vi "Process Data.vi"(7 "AdasLvTemplate in":refnum<class "AdasLvTemplate.lvclass">, 8 "error in":errorcluster, 11 "Node in":refnum<class "AMS Climate Chamber Template.lvclass">) -> (0 "error out":errorcluster, 3 "Node out":refnum<class "AMS Climate Chamber Template.lvclass">, 5 "AdasLvTemplate out":refnum<class "AdasLvTemplate.lvclass">)   [LabVIEW 2023, in "AMS Climate Chamber Template.lvlib" / "AMS Climate Chamber Template.lvclass"]
uses:
  AMS Climate Chamber Template.lvclass
  <vilib>/ADAS Replay HIL/ADAS Plugin Utilities/AdasLvTemplate/AdasLvTemplate.lvclass
  AMS Climate Chamber Template.lvclass/AMS Climate Chamber Template.ctl
  C:/Program Files/National Instruments/AMS plugin/Capabilities/Capabilities/High Level Capabilities/Climate Chamber Cluster/Producer Control.ctl
  C:/Program Files/National Instruments/AMS plugin/Capabilities/Capabilities/High Level Capabilities/Climate Chamber Cluster/Producer Ch.ctl
  C:/Program Files/National Instruments/AMS plugin/Capabilities/Capabilities/High Level Capabilities/Climate Chamber Cluster/Climate Chamber Cluster.lvclass
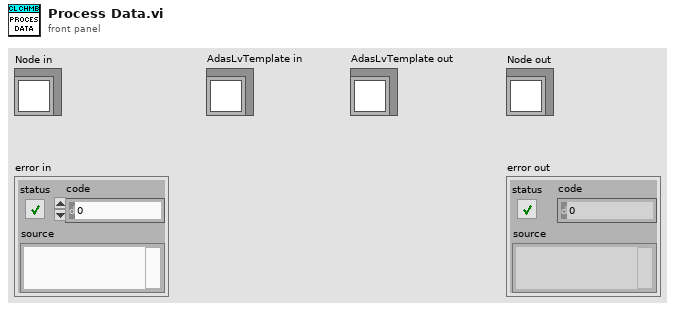
[diagram p1: front panel]
types:
  T1 = typedef "AMS Climate Chamber Template.lvlib/AMS Climate Chamber Template.lvclass/Configuration Params.ctl" = cluster{"Common":T2, "Amount of Channels":u32, "Address":string}
  T2 = typedef "Template Node.lvlib/Template Node.lvclass/Common Configuration Params.ctl" = cluster{"Iteration Interval (s)":dbl, "T0 (ns)":u64, "Priority":i32, "Processor":i32, "Wait in Ready State":bool}
  T3 = typedef "Climate Chamber Cluster.lvclass/Consumer Ch.ctl" = cluster{"Temperature.SP":dbl, "TemperatureMIN.SP":dbl, "TemperatureMAX.SP":dbl, "TemperatureGrad.SP":dbl, "Humidity.SP":dbl, "HumidityMIN.SP":dbl, "HumidityMAX.SP":dbl, "HumidityGrad.SP":dbl}
  T4 = typedef "Climate Chamber Cluster.lvclass/Consumer Control.ctl" = cluster{"OnOff.ACT":bool, "ErrorAcknowledge.ACT":bool}
  T5 = typedef "Climate Chamber Cluster.lvclass/Producer Control.ctl" = cluster{"OnOff.STS":i32, "Error.STS":i32, "Watchdog.STS":i32}
  T6 = typedef "Climate Chamber Cluster.lvclass/Producer Ch.ctl" = cluster{"Temperature.AV":dbl, "Humidity.AV":dbl}
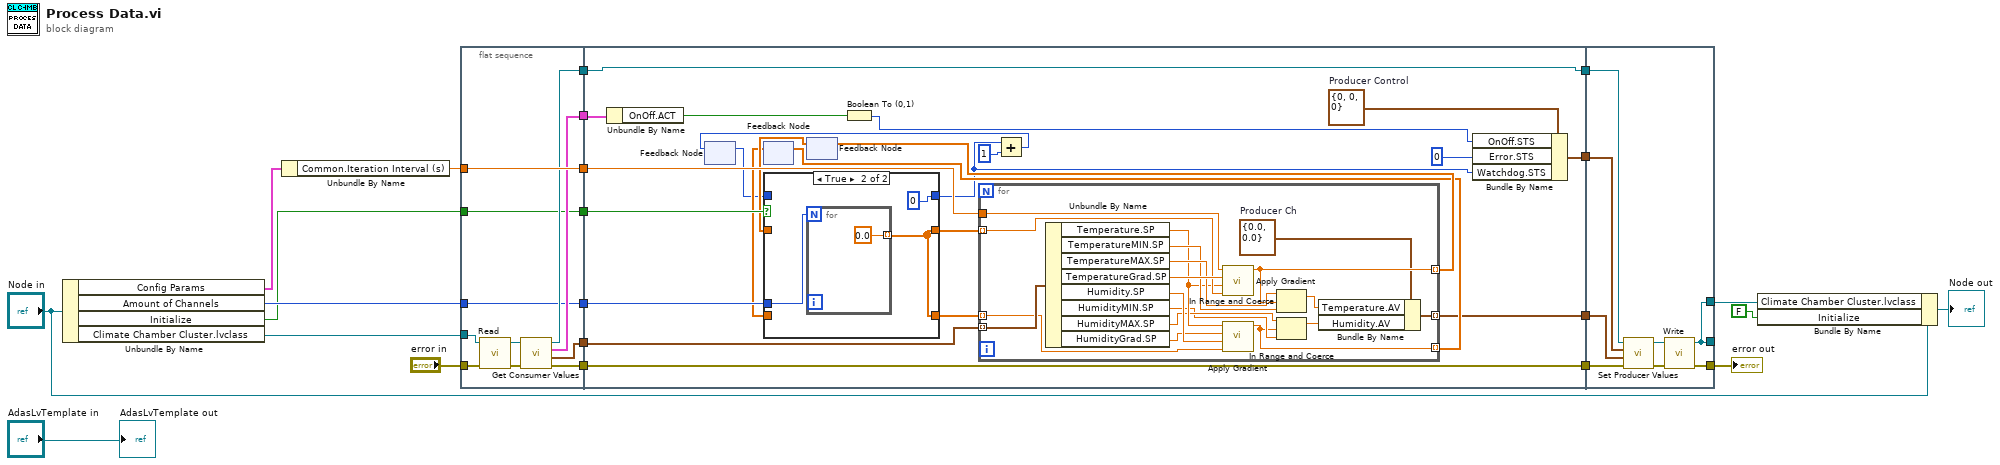
[diagram p0: block diagram]
diagram:
  n1 = Unbundle By Name("Node in") -> ("Config Params"=w22:T1, "Amount of Channels"=w5:u32, "Initialize"=w4:bool, "Climate Chamber Cluster.lvclass"=w1:refnum<class "Climate Chamber Cluster.lvclass">)
  n2 = Unbundle By Name(w22) -> ("Common.Iteration Interval (s)"=w13:dbl)
  n3 = flat-sequence {
    tunnel: w1 -> [w34]
    tunnel: [w28] -> w21
    tunnel: [w31] -> w20
    tunnel: "error in" -> [w33]
    tunnel: [w26] -> w15
    tunnel: [w30] -> w14
    tunnel: w13 -> [w32]
    tunnel: [w32] -> w12
    tunnel: w5 -> [w25]
    tunnel: w4 -> [w24]
    tunnel: [w25] -> w3
    tunnel: [w24] -> w2
    tunnel: w21 -> [w50]
    tunnel: w20 -> [w57]
    tunnel: [w51] -> w19
    tunnel: [w50] -> w18
    tunnel: [w49] -> w16
    tunnel: w15 -> [w49]
    tunnel: w14 -> [w43]
    tunnel: w12 -> [w48]
    tunnel: [w45] -> w11
    tunnel: w3 -> [w42]
    tunnel: w2 -> [w41]
    tunnel: w19 -> [w83]
    tunnel: w18 -> [w85]
    tunnel: w16 -> [w87]
    tunnel: [w90] -> w10
    tunnel: [w89] -> _
    tunnel: w11 -> [w86]
    tunnel: [w89] -> w8
    frame #0 {
      n4 = call-dynamic "Read.vi"("error in"=w33, "Climate Chamber Cluster.lvclass in"=w34) -> ("error out"=w27:errorcluster, "Climate Chamber Cluster.lvclass out"=w29:refnum<class "Climate Chamber Cluster.lvclass">)  [unwired: 8 in]
      n5 = call "Get Consumer Values.vi"("error in"=w27, "Climate Chamber Cluster.lvclass in"=w29) -> ("error out"=w26:errorcluster, "Consumer Ch"=w30:T3[], "Consumer Control"=w31:T4, "Climate Chamber Cluster.lvclass out"=w28:refnum<class "Climate Chamber Cluster.lvclass">)  [unwired: 6 in]
    }
    frame #1 {
      w56 = T5 {"OnOff.STS"=0, "Error.STS"=0, "Watchdog.STS"=0}  # Producer Control
      n6 = Unbundle By Name(w57) -> ("OnOff.ACT"=w55:bool)
      n7 = feedback #1() -> (w35:u16)  [unwired: 1 in]
      n8 = feedback #2() -> (w38:dbl[])  [unwired: 1 in]
      n9 = feedback #3() -> (w40:dbl[])  [unwired: 1 in]
      n10 = case shown="True" w41 {
        tunnel: [w60 w62] -> w39
        tunnel: w42 -> [_ w63]
        tunnel: w40 -> [w60 _]
        tunnel: w38 -> [w59 _]
        tunnel: [w59 w62] -> w37
        tunnel: [w58 u16 0] -> w36
        tunnel: w35 -> [w58 _]
        frame False {
        }
        frame True {
          n11 = for {
            N: w63 -> [_]
            tunnel: [0.0 ("Current Setpoint")] -> w62 mode=indexing
          }
        }
      }
      n12 = Boolean To (0,1)(Boolean=w55) -> (0, 1=w54:i16)
      n13 = for {
        tunnel: w43 -> [w82] mode=indexing
        tunnel: w48 -> [w81]
        tunnel: w39 -> [w77] mode=indexing
        tunnel: [w76] -> w47 mode=indexing
        tunnel: [w70] -> w46 mode=indexing
        tunnel: w37 -> [w69] mode=indexing
        tunnel: [w65] -> w45 mode=indexing
        w68 = T6 {"Temperature.AV"=0.0, "Humidity.AV"=0.0}  # Producer Ch
        n14 = Unbundle By Name(w82) -> ("Temperature.SP"=w73:dbl, "TemperatureMIN.SP"=w78:dbl, "TemperatureMAX.SP"=w79:dbl, "TemperatureGrad.SP"=w80:dbl, "Humidity.SP"=w75:dbl, "HumidityMIN.SP"=w71:dbl, "HumidityMAX.SP"=w72:dbl, "HumidityGrad.SP"=w74:dbl)
        n15 = call "Apply Gradient.vi"("Reminder"=w77, "Setpoint"=w73, "Gradient"=w80, "Iteration Interval"=w81) -> ("Current Setpoint"=w76:dbl)  [unwired: 7 in]
        n16 = call "Apply Gradient.vi"("Reminder"=w69, "Setpoint"=w75, "Gradient"=w74, "Iteration Interval"=w73) -> ("Current Setpoint"=w70:dbl)  [unwired: 7 in]
        n17 = In Range and Coerce(upper limit=w79, x=w76, lower limit=w78) -> (coerced(x)=w67:dbl)  [unwired: 1 out]
        n18 = In Range and Coerce(upper limit=w72, x=w70, lower limit=w71) -> (coerced(x)=w66:dbl)  [unwired: 1 out]
        n19 = Bundle By Name(cluster=w68, "Temperature.AV"=w67, "Humidity.AV"=w66) -> (w65:T6)
      }
      n20 = feedback-in #2(w46) -> ()
      n21 = feedback-in #3(w47) -> ()
      n22 = Add(x=w36, y=u16 1) -> (x+y=w52:u16)
      n23 = feedback-in #1(w52) -> ()
      n24 = Bundle By Name(cluster=w56, "OnOff.STS"=w54, "Error.STS"=0, "Watchdog.STS"=w36) -> (w51:T5)
    }
    frame #2 {
      n25 = call "Set Producer Values.vi"("error in"=w87, "Producer Ch"=w86, "Producer Control"=w83, "Climate Chamber Cluster.lvclass in"=w85) -> ("error out"=w88:errorcluster, "Climate Chamber Cluster.lvclass out"=w84:refnum<class "Climate Chamber Cluster.lvclass">)  [unwired: 6 in]
      n26 = call-dynamic "Write.vi"("error in"=w88, "Climate Chamber Cluster.lvclass in"=w84) -> ("error out"=w90:errorcluster, "Climate Chamber Cluster.lvclass out"=w89:refnum<class "Climate Chamber Cluster.lvclass">)  [unwired: 8 in]
    }
  }
  n27 = Bundle By Name(cluster="Node in", "Climate Chamber Cluster.lvclass"=w8, "Initialize"=FALSE) -> (→"Node out":refnum<class "AMS Climate Chamber Template.lvclass">)
  "error out" <- w10
  "AdasLvTemplate out" <- "AdasLvTemplate in"
